vi "Write String.vi"(6 "error in (no error)":errorcluster, 7 "Bus In":refnum<class "Bus.lvclass">, 8 "Channel Name":string, 9 "Data Value Engineering":dbl, 10 "Data Value Native":dbl, 11 "NI Digital in":refnum<class "No Output.lvclass">) -> (0 "error out":errorcluster, 3 "NI Digital out":refnum<class "No Output.lvclass">, 5 "Bus Out":refnum<class "Bus.lvclass">)   [LabVIEW 2018, in "No Output.lvclass"]
doc: "No Output.lvclass:Read String.vi\n\nThis is the Read String VI forthe No Output class.\n\nInstrument Communication Module Version 1.0\nOctober, 2020 Original Code Consulting Davita Bird\n www.originalcode.com"
uses:
  No Output.lvclass
  Bus/Bus.lvclass
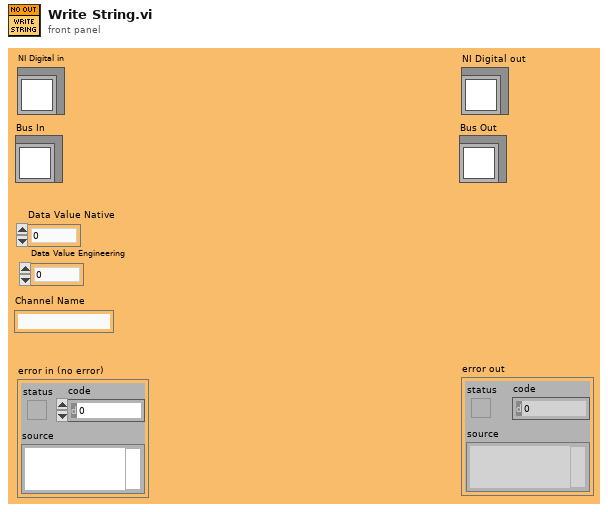
[diagram p1: front panel]
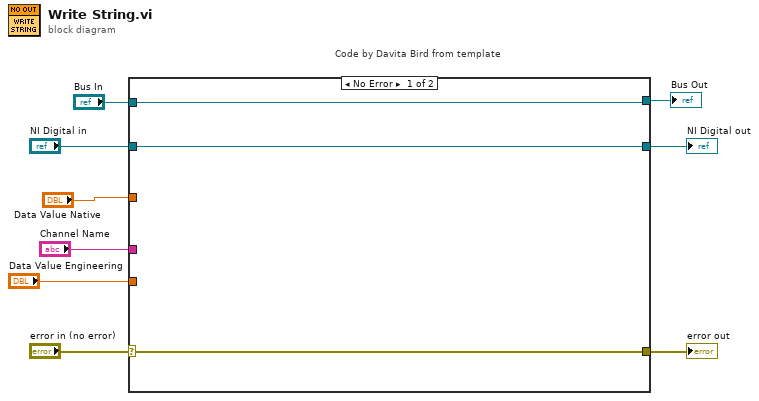
[diagram p0: block diagram]
diagram:
  n1 = case "Code by Davita Bird from template" shown="No Error" "error in (no error)" {
    selector: "error in (no error)" -> [w10 w15]
    tunnel: [w10 w15] -> w8
    tunnel: [w12 w14] -> w7
    tunnel: "NI Digital in" -> [w12 w14]
    tunnel: "Data Value Native" -> [_ _]
    tunnel: "Bus In" -> [w11 w13]
    tunnel: [w11 w13] -> w4
    tunnel: "Channel Name" -> [_ _]
    tunnel: "Data Value Engineering" -> [_ _]
    frame No Error {
    }
    frame Error {
    }
  }
  "error out" <- w8
  "NI Digital out" <- w7
  "Bus Out" <- w4
